vi "Display Data to Table.vi"(11 "Macro":T1) -> (1 "Metadata":string, 3 "Macro Steps":string[][](array[string]))   [LabVIEW 2020, in "MacroAssert.lvlib"]
doc: "Converts <B>Macro</B> to a table of macro steps and a string of associated metadata."
uses:
  MacroAssert.lvlib
  CTLs/Step Type V3.ctl
  CTLs/Step V3.ctl
  CTLs/Macro Cluster V3.ctl
  CTLs/Macro Config V3.ctl
  CTLs/Assertion Type.ctl
panel:
  in  "Virtual Key":u8(ring)=65
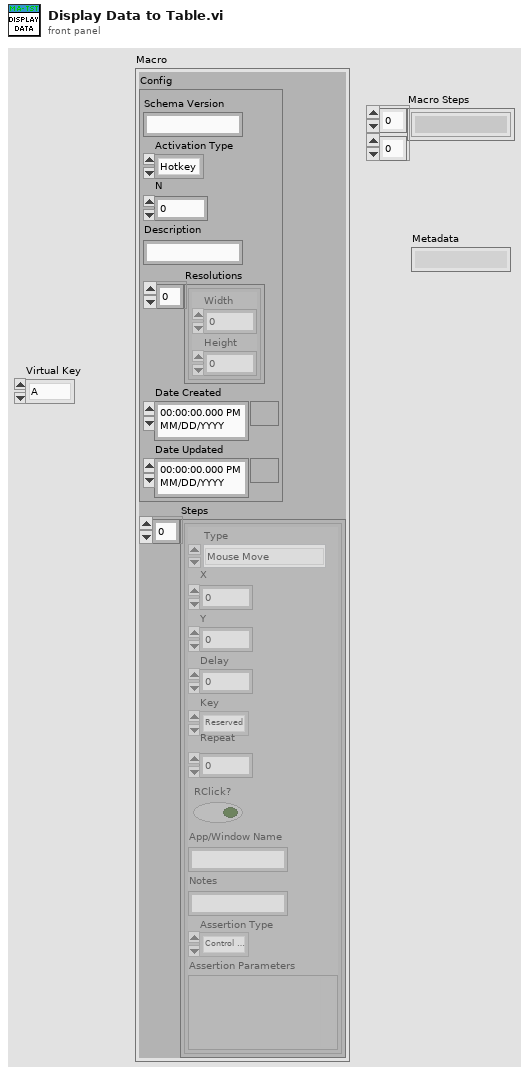
[diagram p1: front panel]
types:
  T1 = typedef "MacroAssert.lvlib/Macro Cluster V3.ctl" = cluster{"Config":T2, "Steps":T3[]}
  T2 = typedef "MacroAssert.lvlib/Macro Config V3.ctl" = cluster{"Schema Version":string, "Activation Type":enum32{"Hotkey", "Automatic"}, "N":i32, "Description":string, "Resolutions":cluster{"Width":i16, "Height":i16}[], "Date Created":timestamp, "Date Updated":timestamp}
  T3 = typedef "MacroAssert.lvlib/Step V3.ctl" = cluster{"Type":T4, "X":i32, "Y":i32, "Delay":i32, "Key":u8, "Repeat":i32, "RClick?":bool, "App/Window Name":string, "Notes":string, "Assertion Type":T5, "Assertion Parameters":variant}
  T4 = typedef "MacroAssert.lvlib/Step Type V3.ctl" = enum16{"Mouse Move", "Mouse Click", "Key Press", "Wait", "Mouse Down", "Mouse Up", "Key Down", "Key Up", "Test Assertion", "Run Application", "Maximize Window", "Restore Window", "Minimize Window", "Close Window", "Bring Window to Front", "Send Window to Back"}
  T5 = typedef "MacroAssert.lvlib/Assertion Type.ctl" = enum16{"Control Position", "Control Visible", "Control Disabled"}
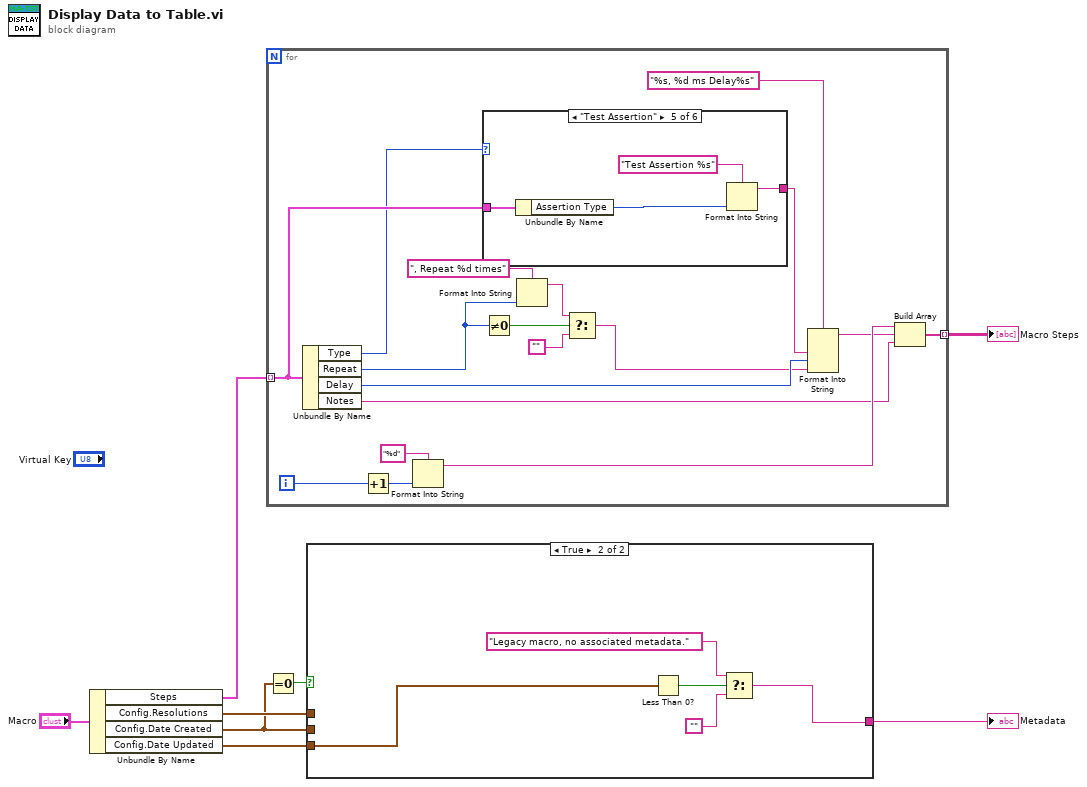
[diagram p0: block diagram]
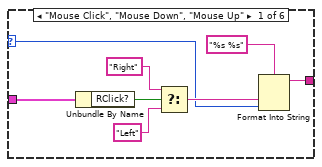
[diagram p2: hidden frame]
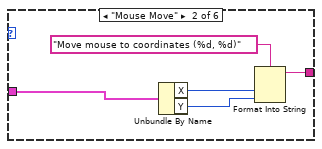
[diagram p3: hidden frame]
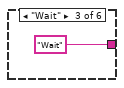
[diagram p4: hidden frame]
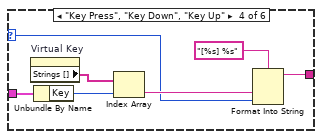
[diagram p5: hidden frame]
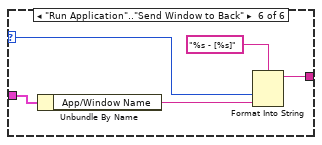
[diagram p6: hidden frame]
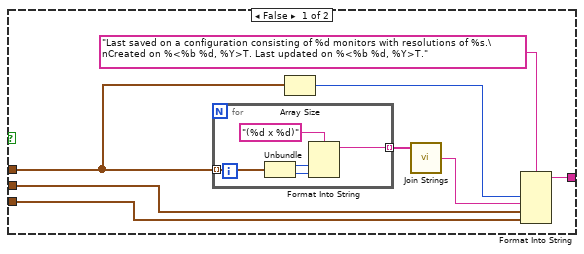
[diagram p7: hidden frame]
diagram:
  n1 = Unbundle By Name("Macro") -> ("Steps"=w6:T3[], "Config.Resolutions"=w4:cluster{"Width":i16, "Height":i16}[], "Config.Date Created"=w1:timestamp, "Config.Date Updated"=w5:timestamp)
  n2 = for {
    tunnel: w6 -> [w25] mode=indexing
    tunnel: [w20] -> w8 mode=indexing
    i -> [w22]
    n3 = Unbundle By Name(w25) -> ("Type"=w11:T4, "Repeat"=w17:i32, "Delay"=w19:i32, "Notes"=w9:string)
    n4 = Increment(x=w22) -> (x+1=w24:i32)
    n5 = Format Into String(format string="%d", w24) -> (resulting string=w21:string)  [unwired: 2 in, 1 out]
    n6 = case shown="\"Test Assertion\"" w11 {
      selector: w11 -> [w28 _ _ w42 _ w54]
      tunnel: w25 -> [w30 w39 _ w47 w51 w56]
      tunnel: [w27 w38 "Wait" w41 w49 w53] -> w12
      frame "Mouse Click", "Mouse Down", "Mouse Up" {
        n7 = Unbundle By Name(w30) -> ("RClick?"=w33:bool)
        n8 = Select(t="Right", s=w33, f="Left") -> (s? t:f=w29:string)
        n9 = Format Into String(format string="%s %s", w29, w28) -> (resulting string=w27:string)  [unwired: 2 in, 1 out]
      }
      frame "Mouse Move" {
        n10 = Unbundle By Name(w39) -> ("X"=w36:i32, "Y"=w35:i32)
        n11 = Format Into String(format string="Move mouse to coordinates (%d, %d)", w36, w35) -> (resulting string=w38:string)  [unwired: 2 in, 1 out]
      }
      frame "Wait" {
      }
      frame "Key Press", "Key Down", "Key Up" {
        n12 = property on="Virtual Key" class="Ring (strict)"() -> ("Strings []"=w45:string[])  [unwired: 2 in, 2 out]
        n13 = Unbundle By Name(w47) -> ("Key"=w44:u8)
        n14 = Index Array(array=w45, index=w44) -> (element=w43:string)
        n15 = Format Into String(format string="[%s] %s", w43, w42) -> (resulting string=w41:string)  [unwired: 2 in, 1 out]
      }
      frame "Test Assertion" {
        n16 = Unbundle By Name(w51) -> ("Assertion Type"=w48:T5)
        n17 = Format Into String(format string="Test Assertion %s", w48) -> (resulting string=w49:string)  [unwired: 2 in, 1 out]
      }
      frame "Run Application".."Send Window to Back" {
        n18 = Unbundle By Name(w56) -> ("App/Window Name"=w52:string)
        n19 = Format Into String(format string="%s - [%s]", w54, w52) -> (resulting string=w53:string)  [unwired: 2 in, 1 out]
      }
    }
    n20 = Not Equal To 0?(x=w17) -> (x != 0?=w16:bool)
    n21 = Format Into String(format string=", Repeat %d times", w17) -> (resulting string=w15:string)  [unwired: 2 in, 1 out]
    n22 = Select(t=w15, s=w16, f="") -> (s? t:f=w13:string)
    n23 = Format Into String(format string="%s, %d ms Delay%s", w12, w19, w13) -> (resulting string=w10:string)  [unwired: 2 in, 1 out]
    n24 = Build Array(w21, w10, w9) -> (w20:string[])
  }
  "Macro Steps" <- w8
  n25 = Equal To 0?(x=w1) -> (x = 0?=w2:bool)
  n26 = case shown="True" w2 {
    tunnel: w5 -> [w63 w74]
    tunnel: w1 -> [w62 _]
    tunnel: w4 -> [w60 _]
    tunnel: [w57 w70] -> w3
    frame False {
      n27 = for {
        tunnel: w60 -> [w68] mode=indexing
        tunnel: [w65] -> w59 mode=indexing
        n28 = Unbundle(w68) -> ("Width"=w66:i16, "Height"=w67:i16)
        n29 = Format Into String(format string="(%d x %d)", w66, w67) -> (resulting string=w65:string)  [unwired: 2 in, 1 out]
      }
      n30 = Array Size(array=w60) -> (size(s)=w61:i32)
      n31 = call <vilib>:"Join Strings.vi"("Strings In"=w59) -> ("String"=w58:string)  [unwired: 2 in]
      n32 = Format Into String(format string="Last saved on a configuration consisting of %d monitors with resolutions of %s.\nCreated on %<%b %d, %Y>T. Last updated on %<%b %d, %Y>T.", w61, w58, w62, w63) -> (resulting string=w57:string)  [unwired: 2 in, 1 out]
    }
    frame True {
      n33 = Less Than 0?(x=w74) -> (x < 0?=w73:bool)
      n34 = Select(t="Legacy macro, no associated metadata.", s=w73, f="") -> (s? t:f=w70:string)
    }
  }
  "Metadata" <- w3
